vi "convert_to_FPGA_parameters.vi"(7 "FPGA clock":dbl=40000000.0, 8 "error in":errorcluster, 11 "All scan parameters":T7={"Fiber parameters"={"Frequency"=100.0, "Amplitude X"=0.0, "Amplitude Y"=0.0, "Initial Amplitude X"=0.0, "Initial Amplitude Y"=0.0, "Phase"=0.0, "Ramp type"=enum."Linear"}, "Spiral parameters"={"Imaging periods"=1.0, "Settling periods"=1.0, "Resting periods"=1.0}, "Run parameters"={"Run mode"=enum."Continuous", "Averages per frame"=1, "No. of frames"=1}, "Acquisition parameters"={"Cycles per pixel"=0, "Image size"=1, "Bidirectional acquisition"=FALSE}, "Fiber parameters pixel_mapper"={"Frequency"=1.0, "Amplitude X"=1.0, "Amplitude Y"=1.0, "Initial Amplitude X"=0.0, "Initial Amplitude Y"=0.0, "Phase"=0.0, "Ramp type"=enum."Linear"}, "Smooth_coeffs_cluster"={"Coeff 1"=0.0, "Coeff 2"=0.0}, "Storage parameters"={"Autosave"=FALSE, "Path"=path ""}, "Mapping corrections"={"Phase increase"=0.0, "Amplitude correction"=0.0}, "Pockels corrections"={"Delay pixels"=0}} {"Pockels corrections"."Delay pixels" min=0 max=10000 step=1; "Mapping corrections"."Phase increase" min=-1.0 max=1.0 step=0.01; "Smooth_coeffs_cluster"."Coeff 1" min=0.0 max=1.0 step=0.05; "Smooth_coeffs_cluster"."Coeff 2" min=0.0 max=1.0 step=0.05; "Fiber parameters pixel_mapper"."Phase" min=-90.0 max=90.0 step=5.0; "Fiber parameters pixel_mapper"."Initial Amplitude Y" min=0.0 max=1.0 step=0.1; "Fiber parameters pixel_mapper"."Initial Amplitude X" min=0.0 max=1.0 step=0.1; "Fiber parameters pixel_mapper"."Amplitude Y" min=0.0 max=4.0 step=0.1; "Fiber parameters pixel_mapper"."Amplitude X" min=0.0 max=4.0 step=0.1; "Fiber parameters pixel_mapper"."Frequency" min=100.0 max=6000.0 step=1.0; "Acquisition parameters"."Image size" items=["128x128 px"=128, "256x256 px"=256, "512x512 px"=512]; "Acquisition parameters"."Cycles per pixel" min=100 max=90000 step=1; "Run parameters"."No. of frames" min=1 max=1000 step=1; "Run parameters"."Averages per frame" min=1 max=32; "Spiral parameters"."Resting periods" min=10.0 max=1000.0 step=1.0; "Spiral parameters"."Settling periods" min=1.0 max=1000.0 step=1.0; "Spiral parameters"."Imaging periods" min=1.0 max=1000.0 step=1.0; "Fiber parameters"."Phase" min=-90.0 max=90.0 step=5.0; "Fiber parameters"."Initial Amplitude Y" min=0.0 max=1.0 step=0.1; "Fiber parameters"."Initial Amplitude X" min=0.0 max=1.0 step=0.1; "Fiber parameters"."Amplitude Y" min=0.0 max=4.0 step=0.1; "Fiber parameters"."Amplitude X" min=0.0 max=4.0 step=0.1; "Fiber parameters"."Frequency" min=100.0 max=6000.0 step=1.0}) -> (0 "error out":errorcluster, 1 "FPGA_acquisition_parameters":T6, 2 "FPGA Scan Parameters":T18={"No. of waveforms"=10, "Continuous scanning"=TRUE}, 3 "FPGA cycle parameters XY":T19, 4 "FPGA ramp parameters XY":T1, 5 "Pixels per spiral":i32=1 min=1 max=90000 step=1)   [LabVIEW 2011, in "Fiberscope_library.lvlib"]
uses:
  Fiberscope_library.lvlib
  fpga/typedefs/cycle_parameters_XY_cluster.ctl
  fpga/typedefs/cycle_parameters_cluster.ctl
  fpga/typedefs/scan_parameters_cluster.ctl
  typedefs/all_scan_parameters_cluster.ctl
  typedefs/fiber_parameters_cluster.ctl
  fpga/typedefs/ramp_type_enum.ctl
  typedefs/spiral_parameters_cluster.ctl
  typedefs/run_parameters_cluster.ctl
  typedefs/run_mode_enum.ctl
  typedefs/acquisition_parameters_cluster.ctl
  typedefs/image_size_I32.ctl
  typedefs/smooth_coeffs_cluster.ctl
  typedefs/storage_parameters_cluster.ctl
  typedefs/mapping_corrections_cluster.ctl
  typedefs/pockels_corrections_cluster.ctl
  typedefs/FPGA_acquisition_parameters.ctl
  fpga/typedefs/ramp_parameters_XY_cluster.ctl
  fpga/typedefs/ramp_parameters_cluster.ctl
  fpga/typedefs/linear_ramp_parameters_cluster.ctl
  fpga/typedefs/sine_ramp_parameters_cluster.ctl
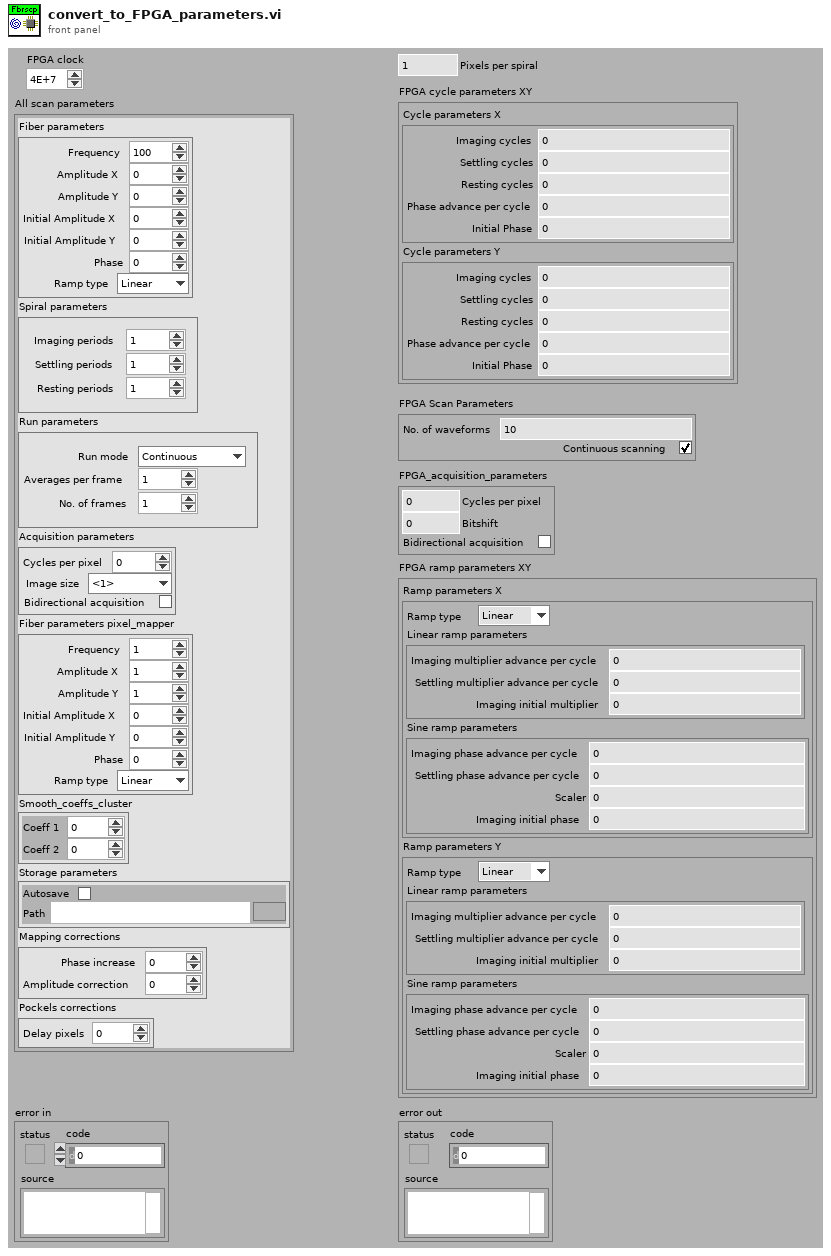
[diagram p1: front panel]
types:
  T1 = typedef "ramp_parameters_XY_cluster.ctl" = cluster{"Ramp parameters X":T2, "Ramp parameters Y":T2}
  T2 = typedef "ramp_parameters_cluster.ctl" = cluster{"Ramp type":T3, "Linear ramp parameters":T4, "Sine ramp parameters":T5}
  T3 = typedef "ramp_type_enum.ctl" = enum8{"Linear", "Sine"}
  T4 = typedef "linear_ramp_parameters_cluster.ctl" = cluster{"Imaging multiplier advance per cycle":fxp<+/-,32,0>, "Settling multiplier advance per cycle":fxp<+/-,32,0>, "Imaging initial multiplier":fxp<+/-,43,12>}
  T5 = typedef "sine_ramp_parameters_cluster.ctl" = cluster{"Imaging phase advance per cycle":fxp<+,32,0>, "Settling phase advance per cycle":fxp<+,32,0>, "Scaler":fxp<+,43,12>, "Imaging initial phase":fxp<+,32,1>}
  T6 = typedef "Fiberscope_library.lvlib/FPGA_acquisition_parameters.ctl" = cluster{"Cycles per pixel":u32, "Bitshift":i8, "Bidirectional acquisition":bool}
  T7 = typedef "Fiberscope_library.lvlib/all_scan_parameters_cluster.ctl" = cluster{"Fiber parameters":T8, "Spiral parameters":T9, "Run parameters":T10, "Acquisition parameters":T12, "Fiber parameters pixel_mapper":T8, "Smooth_coeffs_cluster":T14, "Storage parameters":T15, "Mapping corrections":T16, "Pockels corrections":T17}
  T8 = typedef "Fiberscope_library.lvlib/fiber_parameters_cluster.ctl" = cluster{"Frequency":dbl, "Amplitude X":dbl, "Amplitude Y":dbl, "Initial Amplitude X":dbl, "Initial Amplitude Y":dbl, "Phase":dbl, "Ramp type":T3}
  T9 = typedef "Fiberscope_library.lvlib/spiral_parameters_cluster.ctl" = cluster{"Imaging periods":dbl, "Settling periods":dbl, "Resting periods":dbl}
  T10 = typedef "Fiberscope_library.lvlib/run_parameters_cluster.ctl" = cluster{"Run mode":T11, "Averages per frame":u8, "No. of frames":u32}
  T11 = typedef "Fiberscope_library.lvlib/run_mode_enum.ctl" = enum16{"Continuous", "Single frame", "No. of frames"}
  T12 = typedef "Fiberscope_library.lvlib/acquisition_parameters_cluster.ctl" = cluster{"Cycles per pixel":u32, "Image size":T13, "Bidirectional acquisition":bool}
  T13 = typedef "Fiberscope_library.lvlib/image_size_I32.ctl" = i32
  T14 = typedef "Fiberscope_library.lvlib/smooth_coeffs_cluster.ctl" = cluster{"Coeff 1":dbl, "Coeff 2":dbl}
  T15 = typedef "Fiberscope_library.lvlib/storage_parameters_cluster.ctl" = cluster{"Autosave":bool, "Path":path}
  T16 = typedef "Fiberscope_library.lvlib/mapping_corrections_cluster.ctl" = cluster{"Phase increase":dbl, "Amplitude correction":dbl}
  T17 = typedef "Fiberscope_library.lvlib/pockels_corrections_cluster.ctl" = cluster{"Delay pixels":i32}
  T18 = typedef "scan_parameters_cluster.ctl" = cluster{"No. of waveforms":u16, "Continuous scanning":bool}
  T19 = typedef "cycle_parameters_XY_cluster.ctl" = cluster{"Cycle parameters X":T20, "Cycle parameters Y":T20}
  T20 = typedef "cycle_parameters_cluster.ctl" = cluster{"Imaging cycles":i32, "Settling cycles":i32, "Resting cycles":i32, "Phase advance per cycle":fxp<+,32,0>, "Initial Phase":fxp<+,32,1>}
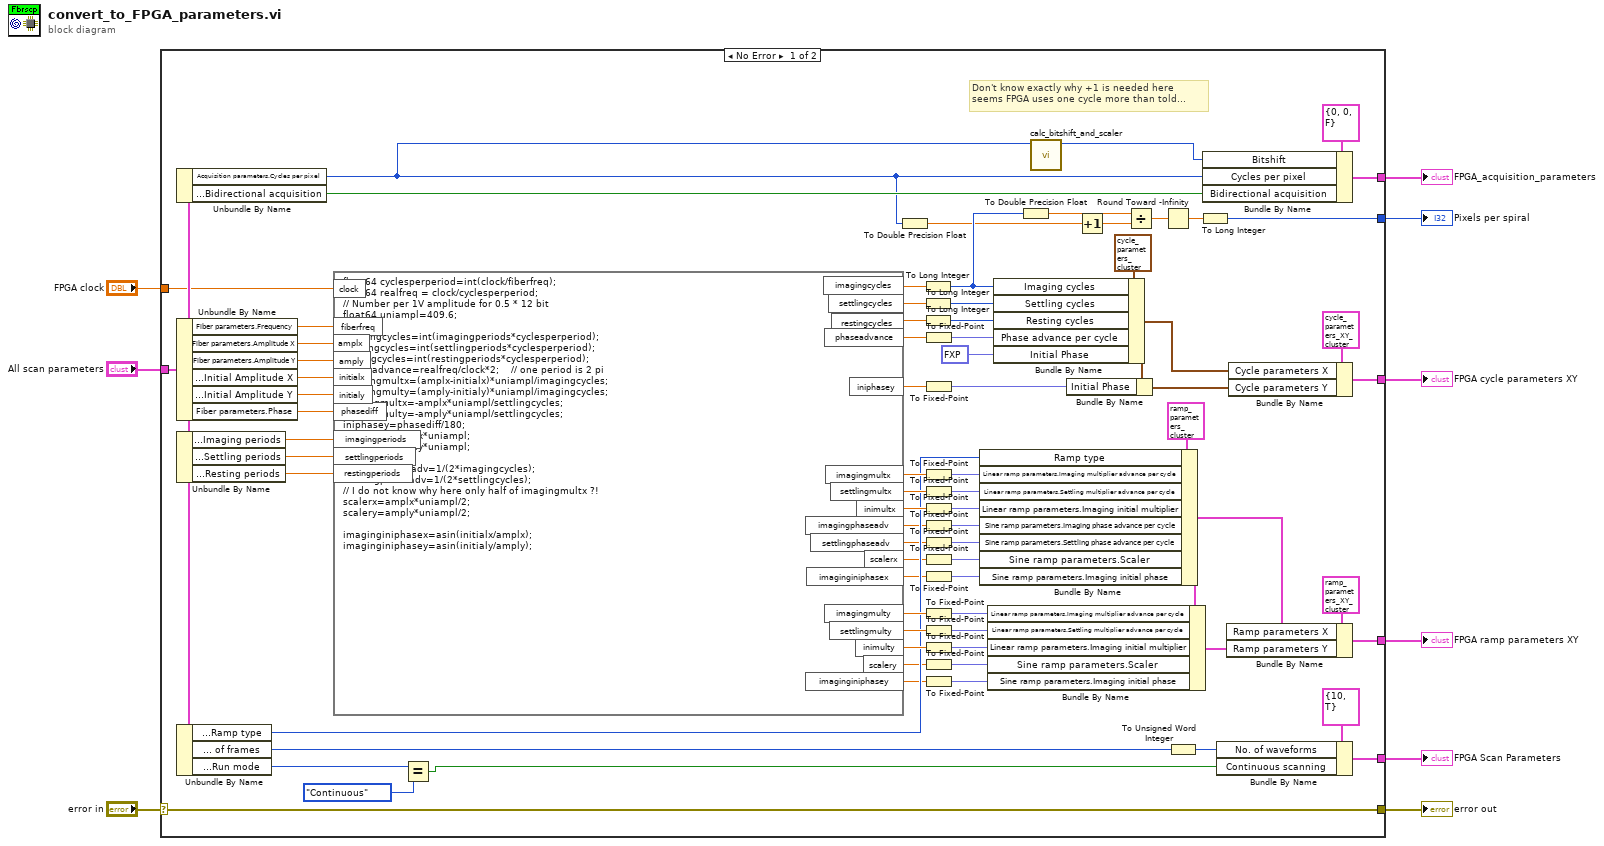
[diagram p0: block diagram]
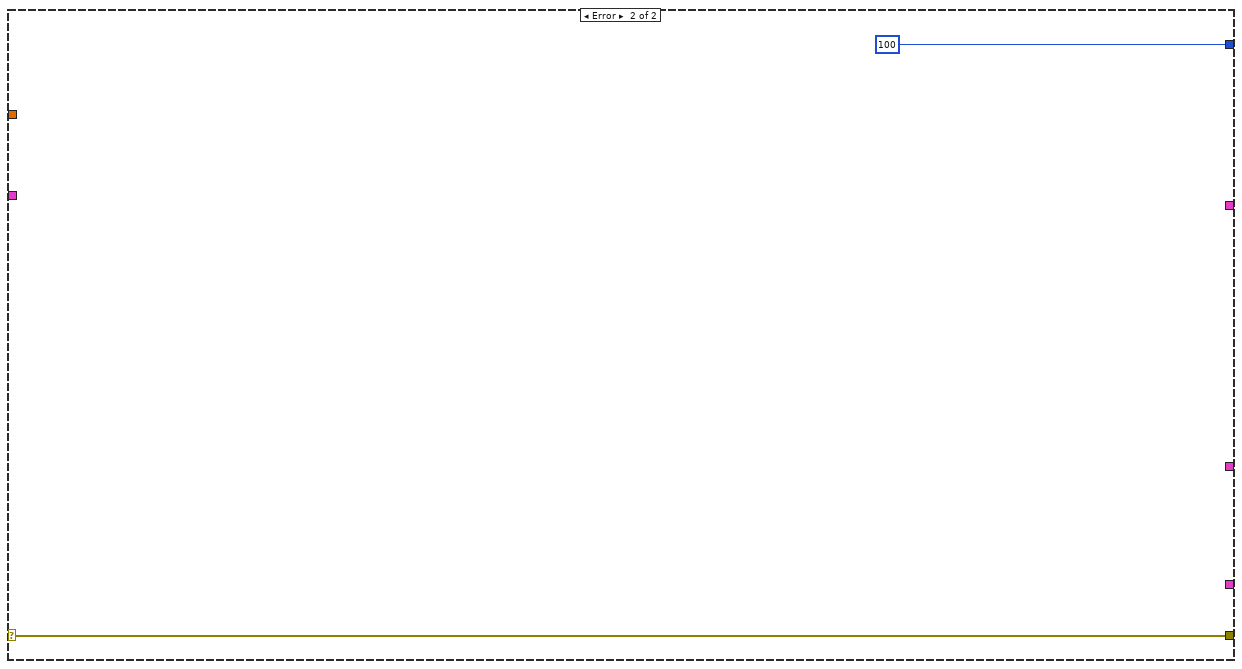
[diagram p2: hidden frame]
diagram:
  n1 = case shown="No Error" "error in" {
    selector: "error in" -> [w85 w87]
    tunnel: [w85 w87] -> w8
    tunnel: [w57 _] -> w7
    tunnel: [w55 _] -> w6
    tunnel: [w49 u32 100] -> w3
    tunnel: "All scan parameters" -> [w46 _]
    tunnel: "FPGA clock" -> [w45 _]
    tunnel: [w43 _] -> w2
    tunnel: [w34 _] -> w1
    frame No Error {
      # "Don't know exactly why +1 is needed here\nseems FPGA uses one cycle more than told..."
      n2 = Unbundle By Name(w46) -> ("Acquisition parameters.Cycles per pixel"=w37:u32, "Acquisition parameters.Bidirectional acquisition"=w38:bool)
      n3 = Unbundle By Name(w46) -> ("Fiber parameters.Frequency"=w84:dbl, "Fiber parameters.Amplitude X"=w83:dbl, "Fiber parameters.Amplitude Y"=w82:dbl, "Fiber parameters.Initial Amplitude X"=w81:dbl, "Fiber parameters.Initial Amplitude Y"=w80:dbl, "Fiber parameters.Phase"=w79:dbl)
      n4 = Unbundle By Name(w46) -> ("Spiral parameters.Imaging periods"=w78:dbl, "Spiral parameters.Settling periods"=w77:dbl, "Spiral parameters.Resting periods"=w76:dbl)
      n5 = Unbundle By Name(w46) -> ("Fiber parameters.Ramp type"=w23:T3, "Run parameters.No. of frames"=w51:u32, "Run parameters.Run mode"=w54:T11)
      n6 = formula code="float64 cyclesperperiod=int(clock/fiberfreq);\nfloat64 realfreq = clock/cyclesperperiod;\n// Number per 1V amplitude for 0.5 * 12 bit\nfloat64 uniampl=409.6;\n\nimagingcycles=int(imagingperiods*cyclesperperiod);\nsettlingcycles=int(settlingperiods*cyclesperperiod);\nrestingcycles=int(restingperiods*cyclesperperiod);\nphaseadvance=realfreq/clock*2;    // one period is 2 pi\nimagingmultx=(amplx-initialx)*uniampl/imagingcycles;\nimagingmulty=(amply-initialy)*uniampl/imagingcycles;\nsettlingmultx=-amplx*uniampl/settlingcycles;\nsettlingmulty=-amply*uniampl/settlingcycles;\niniphasey=phasediff/180;\ninimultx=initialx*uniampl;\ninimulty=initialy*uniampl;\n\nimagingphaseadv=1/(2*imagingcycles);\nsettlingphaseadv=1/(2*settlingcycles);\n// I do not know why here only half of imagingmultx ?!\nscalerx=amplx*uniampl/2;\nscalery=amply*uniampl/2;\n\nimaginginiphasex=asin(initialx/amplx);\nimaginginiphasey=asin(initialy/amply);"("fiberfreq"=w84, "imagingperiods"=w78, "settlingperiods"=w77, "restingperiods"=w76, "amplx"=w83, "amply"=w82, "phasediff"=w79, "initialx"=w81, "initialy"=w80, "clock"=w45) -> ("imagingcycles"=w74:dbl, "settlingcycles"=w73:dbl, "restingcycles"=w71:dbl, "phaseadvance"=w69:dbl, "imagingmultx"=w67:dbl, "imagingmulty"=w62:dbl, "iniphasey"=w58:dbl, "inimultx"=w65:dbl, "inimulty"=w60:dbl, "settlingmultx"=w66:dbl, "settlingmulty"=w61:dbl, "imagingphaseadv"=w22:dbl, "settlingphaseadv"=w20:dbl, "scalerx"=w18:dbl, "imaginginiphasex"=w16:dbl, "scalery"=w12:dbl, "imaginginiphasey"=w11:dbl)
      n7 = Equal?(x=w54, y=run_mode_enum."Continuous") -> (x = y?=w52:bool)
      n8 = To Double Precision Float(number=w37) -> (double precision float=w36:dbl)
      n9 = To Long Integer(number=w74) -> (32bit integer=w48:i32)
      n10 = To Long Integer(number=w73) -> (32bit integer=w72:i32)
      n11 = To Long Integer(number=w71) -> (32bit integer=w70:i32)
      n12 = To Fixed-Point(number=w69) -> (fixed-point=w68:fxp<+,32,0>)  [unwired: 1 in]
      n13 = To Fixed-Point(number=w58) -> (fixed-point=w59:fxp<+,32,1>)  [unwired: 1 in]
      n14 = To Fixed-Point(number=w67) -> (fixed-point=w33:fxp<+/-,32,0>)  [unwired: 1 in]
      n15 = To Fixed-Point(number=w66) -> (fixed-point=w32:fxp<+/-,32,0>)  [unwired: 1 in]
      n16 = To Fixed-Point(number=w65) -> (fixed-point=w31:fxp<+/-,43,12>)  [unwired: 1 in]
      n17 = To Fixed-Point(number=w22) -> (fixed-point=w21:fxp<+,32,0>)  [unwired: 1 in]
      n18 = To Fixed-Point(number=w20) -> (fixed-point=w19:fxp<+,32,0>)  [unwired: 1 in]
      n19 = To Fixed-Point(number=w18) -> (fixed-point=w17:fxp<+,43,12>)  [unwired: 1 in]
      n20 = To Fixed-Point(number=w16) -> (fixed-point=w15:fxp<+,32,1>)  [unwired: 1 in]
      n21 = To Fixed-Point(number=w62) -> (fixed-point=w29:fxp<+/-,32,0>)  [unwired: 1 in]
      n22 = To Fixed-Point(number=w61) -> (fixed-point=w28:fxp<+/-,32,0>)  [unwired: 1 in]
      n23 = To Fixed-Point(number=w60) -> (fixed-point=w27:fxp<+/-,43,12>)  [unwired: 1 in]
      n24 = To Fixed-Point(number=w12) -> (fixed-point=w14:fxp<+,43,12>)  [unwired: 1 in]
      n25 = To Fixed-Point(number=w11) -> (fixed-point=w13:fxp<+,32,1>)  [unwired: 1 in]
      n26 = Bundle By Name(cluster=T2 {"Ramp type"=enum."Linear", "Linear ramp parameters"={"Imaging multiplier advance per cycle"=0.0, "Settling multiplier advance per cycle"=0.0, "Imaging initial multiplier"=0.0}, "Sine ramp parameters"={"Imaging phase advance per cycle"=0.0, "Settling phase advance per cycle"=0.0, "Scaler"=0.0, "Imaging initial phase"=0.0}} ("Ramp parameters"), "Ramp type"=w23, "Linear ramp parameters.Imaging multiplier advance per cycle"=w33, "Linear ramp parameters.Settling multiplier advance per cycle"=w32, "Linear ramp parameters.Imaging initial multiplier"=w31, "Sine ramp parameters.Imaging phase advance per cycle"=w21, "Sine ramp parameters.Settling phase advance per cycle"=w19, "Sine ramp parameters.Scaler"=w17, "Sine ramp parameters.Imaging initial phase"=w15) -> (w10:T2)
      n27 = Bundle By Name(cluster=w10, "Linear ramp parameters.Imaging multiplier advance per cycle"=w29, "Linear ramp parameters.Settling multiplier advance per cycle"=w28, "Linear ramp parameters.Imaging initial multiplier"=w27, "Sine ramp parameters.Scaler"=w14, "Sine ramp parameters.Imaging initial phase"=w13) -> (w24:T2)
      n28 = Bundle By Name(cluster=T20 {"Imaging cycles"=0, "Settling cycles"=0, "Resting cycles"=0, "Phase advance per cycle"=0.0, "Initial Phase"=0.0} ("FPGA Cycle Parameters Y"), "Imaging cycles"=w48, "Settling cycles"=w72, "Resting cycles"=w70, "Phase advance per cycle"=w68, "Initial Phase"=fxp<+,32,1> 0.0) -> (w26:T20)
      n29 = To Double Precision Float(number=w48) -> (double precision float=w47:dbl)
      n30 = call "calc_bitshift_and_scaler.vi"("Cycles per pixel"=w37) -> ("Bitshift"=w42:i8)  [unwired: 8 in, 2 out]
      n31 = Bundle By Name(cluster=w26, "Initial Phase"=w59) -> (w25:T20)
      n32 = Increment(x=w36) -> (x+1=w39:dbl)
      n33 = Divide(x=w47, y=w39) -> (x/y=w41:dbl)
      n34 = Round Toward -Infinity(1:w41) -> (0:w40:dbl)
      n35 = To Unsigned Word Integer(number=w51) -> (unsigned 16bit integer=w50:u16)
      n36 = To Long Integer(number=w40) -> (32bit integer=w49:i32)
      n37 = Bundle By Name(cluster=T6 {"Cycles per pixel"=0, "Bitshift"=0, "Bidirectional acquisition"=FALSE} ("FPGA_acquisition_parameters 2"), "Bitshift"=w42, "Cycles per pixel"=w37, "Bidirectional acquisition"=w38) -> (w43:T6)
      n38 = Bundle By Name(cluster=T18 {"No. of waveforms"=10, "Continuous scanning"=TRUE} ("FPGA Scan Parameters"), "No. of waveforms"=w50, "Continuous scanning"=w52) -> (w55:T18)
      n39 = Bundle By Name(cluster=T1 {"Ramp parameters X"={"Ramp type"=enum."Linear", "Linear ramp parameters"={"Imaging multiplier advance per cycle"=0.0, "Settling multiplier advance per cycle"=0.0, "Imaging initial multiplier"=0.0}, "Sine ramp parameters"={"Imaging phase advance per cycle"=0.0, "Settling phase advance per cycle"=0.0, "Scaler"=0.0, "Imaging initial phase"=0.0}}, "Ramp parameters Y"={"Ramp type"=enum."Linear", "Linear ramp parameters"={"Imaging multiplier advance per cycle"=0.0, "Settling multiplier advance per cycle"=0.0, "Imaging initial multiplier"=0.0}, "Sine ramp parameters"={"Imaging phase advance per cycle"=0.0, "Settling phase advance per cycle"=0.0, "Scaler"=0.0, "Imaging initial phase"=0.0}}} ("Ramp parameters XY"), "Ramp parameters X"=w10, "Ramp parameters Y"=w24) -> (w34:T1)
      n40 = Bundle By Name(cluster=T19 {"Cycle parameters X"={"Imaging cycles"=0, "Settling cycles"=0, "Resting cycles"=0, "Phase advance per cycle"=0.0, "Initial Phase"=0.0}, "Cycle parameters Y"={"Imaging cycles"=0, "Settling cycles"=0, "Resting cycles"=0, "Phase advance per cycle"=0.0, "Initial Phase"=0.0}} ("FPGA Cycle Parameters XY"), "Cycle parameters X"=w26, "Cycle parameters Y"=w25) -> (w57:T19)
    }
    frame Error {
    }
  }
  "error out" <- w8
  "FPGA cycle parameters XY" <- w7
  "FPGA Scan Parameters" <- w6
  "Pixels per spiral" <- w3
  "FPGA_acquisition_parameters" <- w2
  "FPGA ramp parameters XY" <- w1
